vi "GetInputCount.vi"(7 "DLL path":path, 8 "error in (no error)":errorcluster, 11 "session id in":i32) -> (0 "error out":errorcluster, 2 "InputCount":i32, 3 "session id out":i32)   [LabVIEW 2017, in "ONNX Class Library.lvlib"]
doc: "/**\n * @brief Получить количество входов модели\n * \n * Возвращает число входных тензоров, которые ожидает модель.\n * Большинство моделей имеют 1 вход, но некоторые (например, мульти-модальные)\n * могут иметь несколько.\n * \n * @param sessionId [IN] ID сессии\n * \n * @return int32: Количество входов (0 или больше)\n * @return int32: 0 если сессия не найдена или не загружена\n */\nint GetInputCount(int sessionId);"
uses:
  ONNX Class Library.lvlib
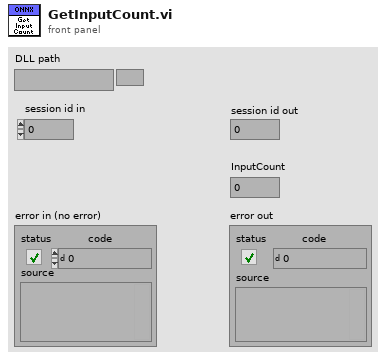
[diagram p1: front panel]
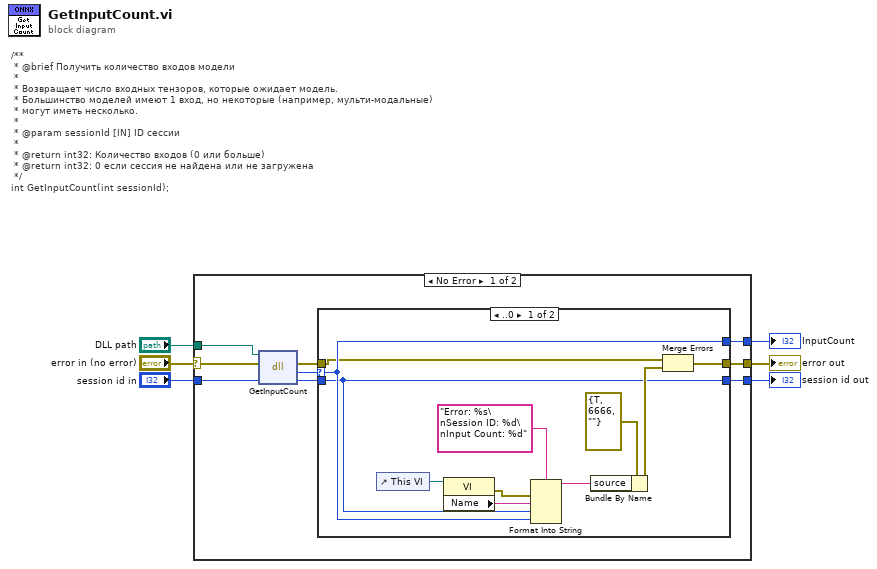
[diagram p0: block diagram]
diagram:
  # "/**\n * @brief Получить количество входов модели\n * \n * Возвращает число входных тензоров, которые ожидает модель.\n * Большинство моделей имеют 1 вход, но некоторые (например, мульти-модальные)\n * могут иметь несколько.\n * \n * @param sessionId [IN] ID сессии\n * \n * @return int32: Количество входов (0 или больше)\n * @return int32: 0 если сессия не найдена или не загружена\n */\nint GetInputCount(int sessionId);"
  n1 = case shown="No Error" "error in (no error)" {
    selector: "error in (no error)" -> [w8 w31]
    tunnel: "session id in" -> [w15 w30]
    tunnel: [w12 w31] -> w5
    tunnel: [w10 w30] -> w4
    tunnel: [w9 _] -> w3
    tunnel: "DLL path" -> [w7 _]
    frame No Error {
      n2 = dll-call lib="home/ivan/LabVIEWData/ONNX/Test/libonnx_wrapper/unix64/libonnx_wrapper.so" fn="GetInputCount"(path in=w7, error in=w8, "sessionId"=w15) -> (error out=w13:errorcluster, "return"=w14:i32, "sessionId"=w11:i32)  [unwired: 1 in, 1 out]
      n3 = case shown="..0" w14 {
        selector: w14 -> [w20 w27]
        tunnel: w13 -> [w16 w29]
        tunnel: [w17 w29] -> w12
        tunnel: w11 -> [w18 w28]
        tunnel: [w18 w28] -> w10
        tunnel: [w20 w27] -> w9
        frame ..0 {
          n4 = control-ref of="This VI"() -> (w23:refnum<vi>)
          n5 = property class="VI"(reference=w23) -> (error out=w19:errorcluster, "Name"=w22:string)  [unwired: 1 in, 1 out]
          n6 = Format Into String(format string="Error: %s\nSession ID: %d\nInput Count: %d", error in=w19, w22, w18, w20) -> (resulting string=w24:string)  [unwired: 1 in, 1 out]
          n7 = Bundle By Name(cluster=errorcluster {"status"=TRUE, "code"=6666, "source"=""} ("error out"), "source"=w24) -> (w25:errorcluster)
          n8 = Merge Errors(w16, w25) -> (w17:errorcluster)
        }
        frame 1.. {
        }
      }
    }
    frame Error {
    }
  }
  "error out" <- w5
  "session id out" <- w4
  "InputCount" <- w3
